vi "Autonomous Independent.vi"() -> ()   [LabVIEW 2012]
doc: "This VI is called when autonomous begins, and will automatically be terminated when autonomous ends. You can carry out timed or sensor driven robot movement independently without needing to return to the caller."
uses:
  <vilib>/Rock Robotics/WPI/DriverStation/WPI_DriverStationMatch Info.ctl
  <vilib>/Rock Robotics/WPI/Solenoid/WPI_SolenoidValue.ctl
  <vilib>/Rock Robotics/WPI/Relay/WPI_RelayValue.ctl
  Robot Global Data.vi
  <vilib>/addons/control/pid/pid.llb/PID (DBL).vi
  <vilib>/Rock Robotics/WPI/Solenoid/WPI_SolenoidSetEnum.vi
  <vilib>/Rock Robotics/WPI/Joystick/WPI_JoystickGetSetRefNum.vi
  <vilib>/addons/control/pid/NI_PID_pid.lvlib
panel:
  out "Reseting constant":bool
  in  "Threshold for shooter":dbl=0.015
  out "Ready To Fire":bool
  in  "PID gains":T1={"proportional gain (Kc)"=1.0, "integral time (Ti, min)"=0.007, "derivative time (Td, min)"=0.0} {"derivative time (Td, min)" format="%.3f"; "integral time (Ti, min)" format="%.3f"; "proportional gain (Kc)" format="%.3f"}
  in  "Maximum Encoder speed":dbl=25000.0
  out "Time Last Fired":dbl
  in  "Posistioned":string="Nothing"
  in  "S On Time":dbl=200.0
  in  "S Off Time":dbl=500.0
  in  "Shooter Speed":dbl format="%.2f"
  in  "Shooter On":bool=TRUE
  in  "Match Info":T2={"Autonomous Elapsed Seconds"=0.0, "TeleOp Elapsed Seconds"=0.0, "Disabled Elapsed Seconds"=0.0, "Visited Autonomous"=FALSE, "Visited TeleOp"=FALSE, "Visited Disabled"=FALSE, "Autonomous Settings"={"Autonomous Style"=enum."Independent", "VI Refnum"=refnum}}
  out "Angle Target":dbl
  out "Distance From Target":dbl
  in  "Current Status":string="Roaming"
  in  "Angle to Move":dbl format="%.2f"
  in  "Feet To Move at Begin":dbl format="%.2f"
  # "Be sure to right-click and choose Data Operations>>Make Current Value default if you want to save the array values with the VI"
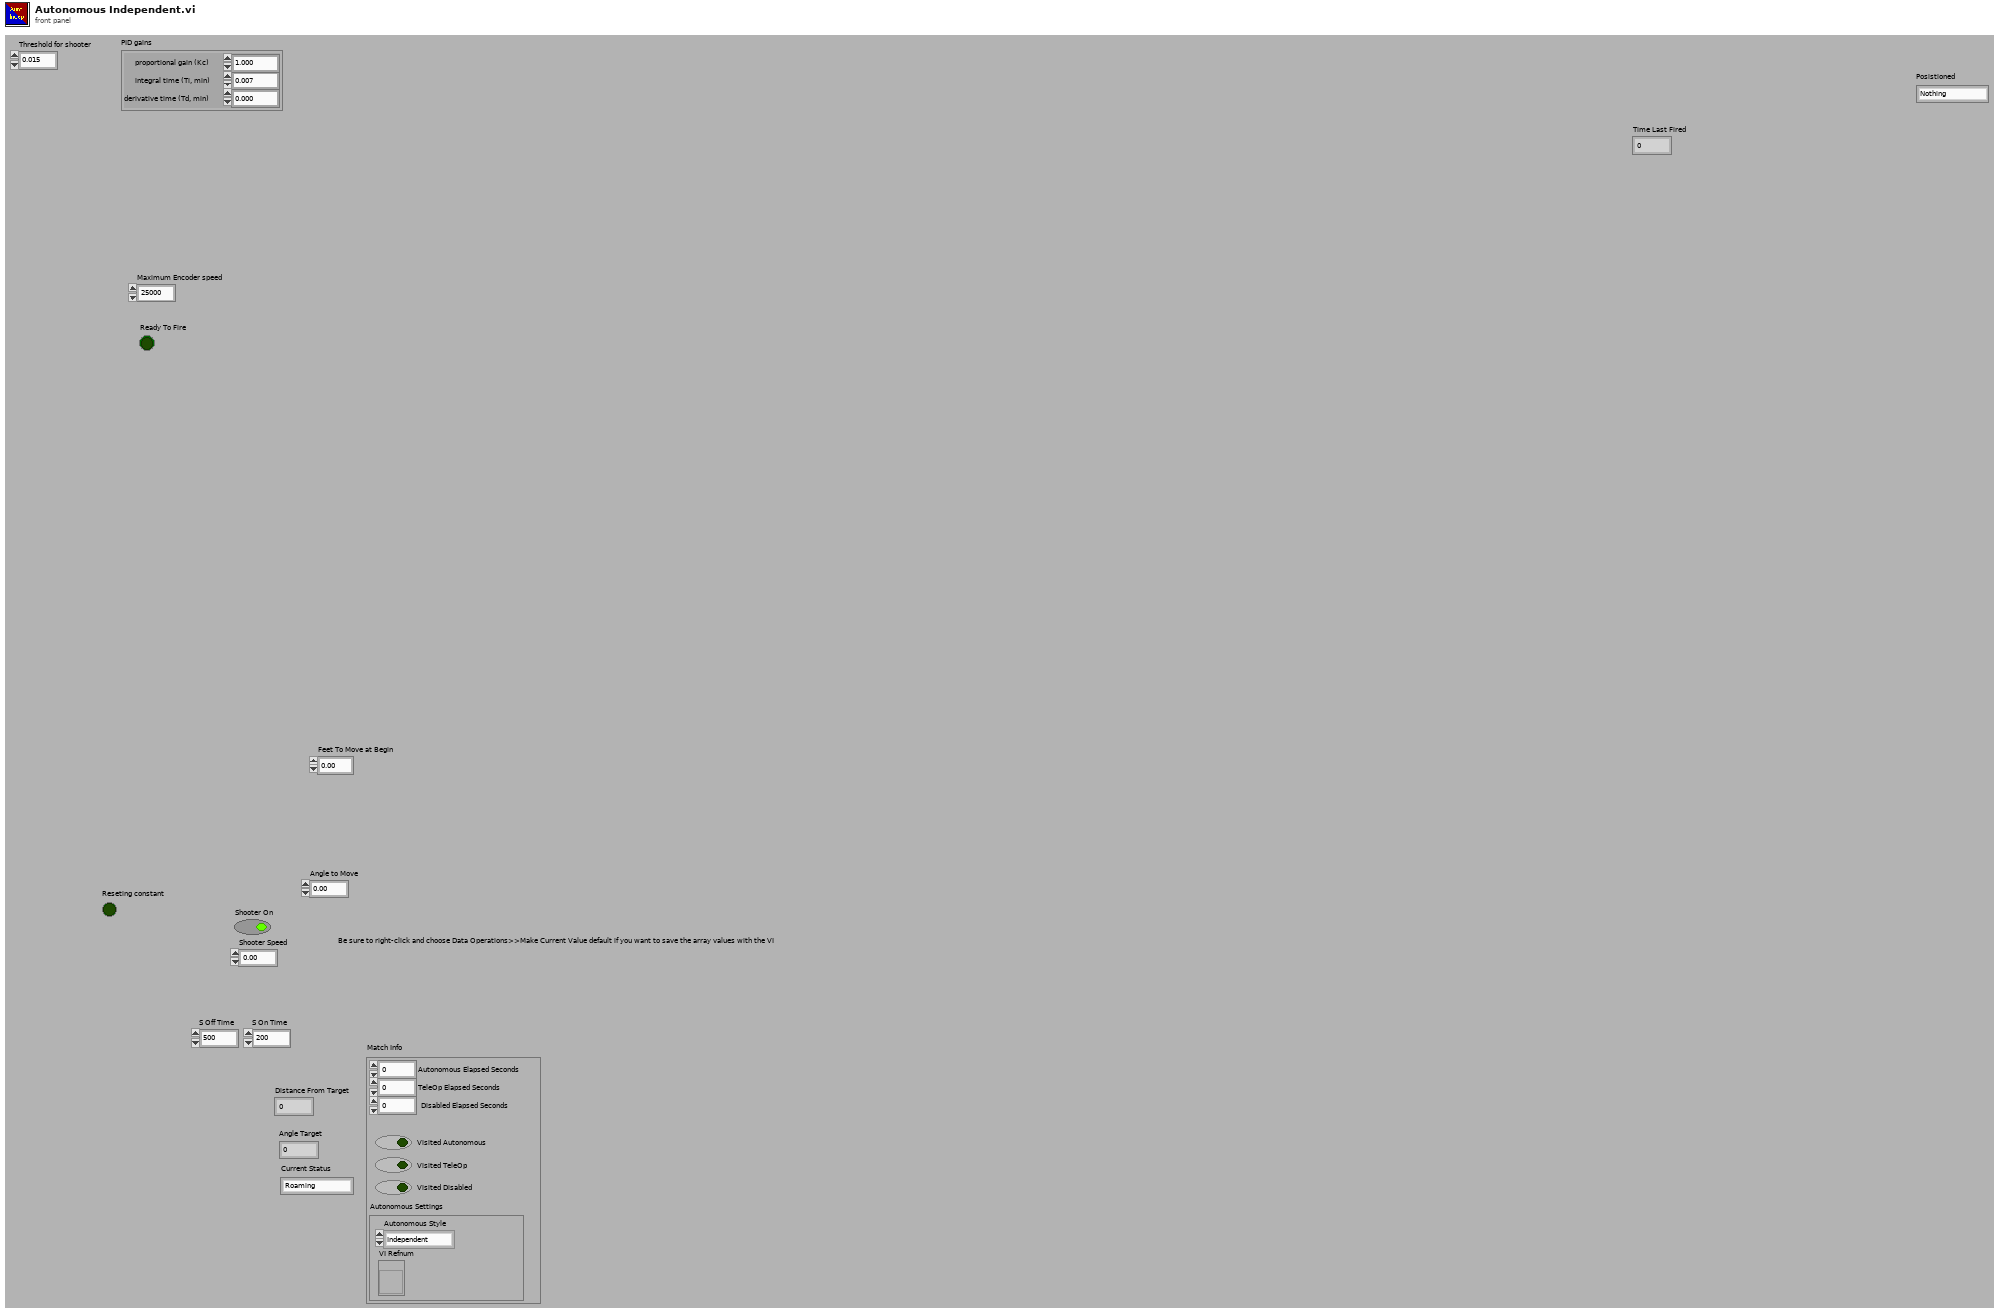
[diagram p1: front panel]
types:
  T1 = cluster{"proportional gain (Kc)":dbl, "integral time (Ti, min)":dbl, "derivative time (Td, min)":dbl}
  T2 = typedef "WPI_DriverStationMatch Info.ctl" = cluster{"Autonomous Elapsed Seconds":dbl, "TeleOp Elapsed Seconds":dbl, "Disabled Elapsed Seconds":dbl, "Visited Autonomous":bool, "Visited TeleOp":bool, "Visited Disabled":bool, "Autonomous Settings":cluster{"Autonomous Style":enum16{"Iterative", "Independent"}, "VI Refnum":refnum<vi>}}
  T3 = typedef "WPI_SolenoidValue.ctl" = enum16{"Off", "On", "Forward", "Reverse"}
  T4 = typedef "WPI_RelayValue.ctl" = enum16{"Off", "On", "Forward", "Reverse"}
  T5 = typedef "WPI_EncoderDevRef.ctl" = cluster{"DevStatus":errorcluster, "EncoderIndex":T6, "CounterIndex":T7, "DistancePerCount":dbl, "Decoding Type":T8}
  T6 = typedef "FPGA_EncoderIdx.ctl" = enum8{"Enc 0", "Enc 1", "Enc 2", "Enc 3", "Invalid"}
  T7 = typedef "FPGA_CounterCtrSystemIndex.ctl" = enum8{"Ctr 0", "Ctr 1", "Ctr 2", "Ctr 3", "Ctr 4", "Ctr 5", "Ctr 6", "Ctr 7", "Invalid"}
  T8 = typedef "WPI_EncoderType.ctl" = enum16{"1x", "2x", "4x"}
  T9 = typedef "WPI_RelayDevRef.ctl" = cluster{"DevStatus":errorcluster, "Relay Channel":T10, "Digital Module":T11, "Relay Direction":T12}
  T10 = typedef "FPGA_DIORelayChannel.ctl" = enum8{"Relay 1", "Relay 2", "Relay 3", "Relay 4", "Relay 5", "Relay 6", "Relay 7", "Relay 8", "Invalid"}
  T11 = typedef "FPGA_TypedefDigitalModule.ctl" = enum16{"Digital Module 1", "Digital Module 2"}
  T12 = typedef "WPI_RelayDirection.ctl" = enum16{"Both directions", "Forward only", "Reverse only"}
  T13 = typedef "WPI_SolenoidDevRef.ctl" = cluster{"DevStatus":errorcluster, "Solenoid Module":T14, "Forward Solenoid Channel":T15, "Reverse Solenoid Channel":T15}
  T14 = typedef "FPGA_TypedefSolenoidModule.ctl" = enum16{"Solenoid Module 1", "Solenoid Module 2"}
  T15 = typedef "WPI_SolenoidChannel.ctl" = enum8{"Solenoid 1", "Solenoid 2", "Solenoid 3", "Solenoid 4", "Solenoid 5", "Solenoid 6", "Solenoid 7", "Solenoid 8", "Invalid"}
  T16 = cluster{"Center Position":cluster{"X":dbl, "Y":dbl}, "Distance (ft)":dbl, "Center":bool}[]
  T17 = cluster{"Center Position":cluster{"X":dbl, "Y":dbl}, "Distance (ft)":dbl, "Center":bool}
  T18 = typedef "WPI_MotorControlDeviceRef.ctl" = cluster{"DeviceStatus":errorcluster, "Type":enum16{"PWM", "CAN"}, "PWM":cluster{"Digital Module":T11, "PWM Channel":T19, "DeadBand":T20}, "CAN":cluster{"Device Number":u8, "Control Mode":T21, "Semaphore":T22, "Max Vout":dbl}, "Invert":bool, "TransformRef":T23, "InvTransformRef":T23}
  T19 = typedef "FPGA_DIOPWMChannel.ctl" = enum8{"PWM 1", "PWM 2", "PWM 3", "PWM 4", "PWM 5", "PWM 6", "PWM 7", "PWM 8", "PWM 9", "PWM 10", "Invalid"}
  T20 = typedef "WPI_PWMDeadband.ctl" = cluster{"Name":string, "maxPositivePwm":i32, "minPositivePwm":i32, "centerPwm":i32, "maxNegativePwm":i32, "minNegativePwm":i32, "angularRange":u16}
  T21 = typedef "WPI_CANJaguar_ControlMode.ctl" = enum8{"Percent VBus", "Current", "Speed", "Position", "Voltage"}
  T22 = typedef "Semaphore RefNum" = refnum<k1>
  T23 = typedef "WPI_PWMTransform_ConPane.ctl" = refnum<vi>
  T24 = typedef "WPI_JoystickDevRef.ctl" = cluster{"Device":T25}
  T25 = typedef "WPI_JoystickDeviceEnum.ctl" = enum16{"USB 1", "USB 2", "USB 3", "USB 4", "Kinect 1", "Kinect 2"}
  T26 = cluster{"axis 1 (x)":dbl, "axis 2 (y)":dbl, "axis 3 (throttle)":dbl, "axis 4":dbl, "axis 5":dbl, "axis 6":dbl}
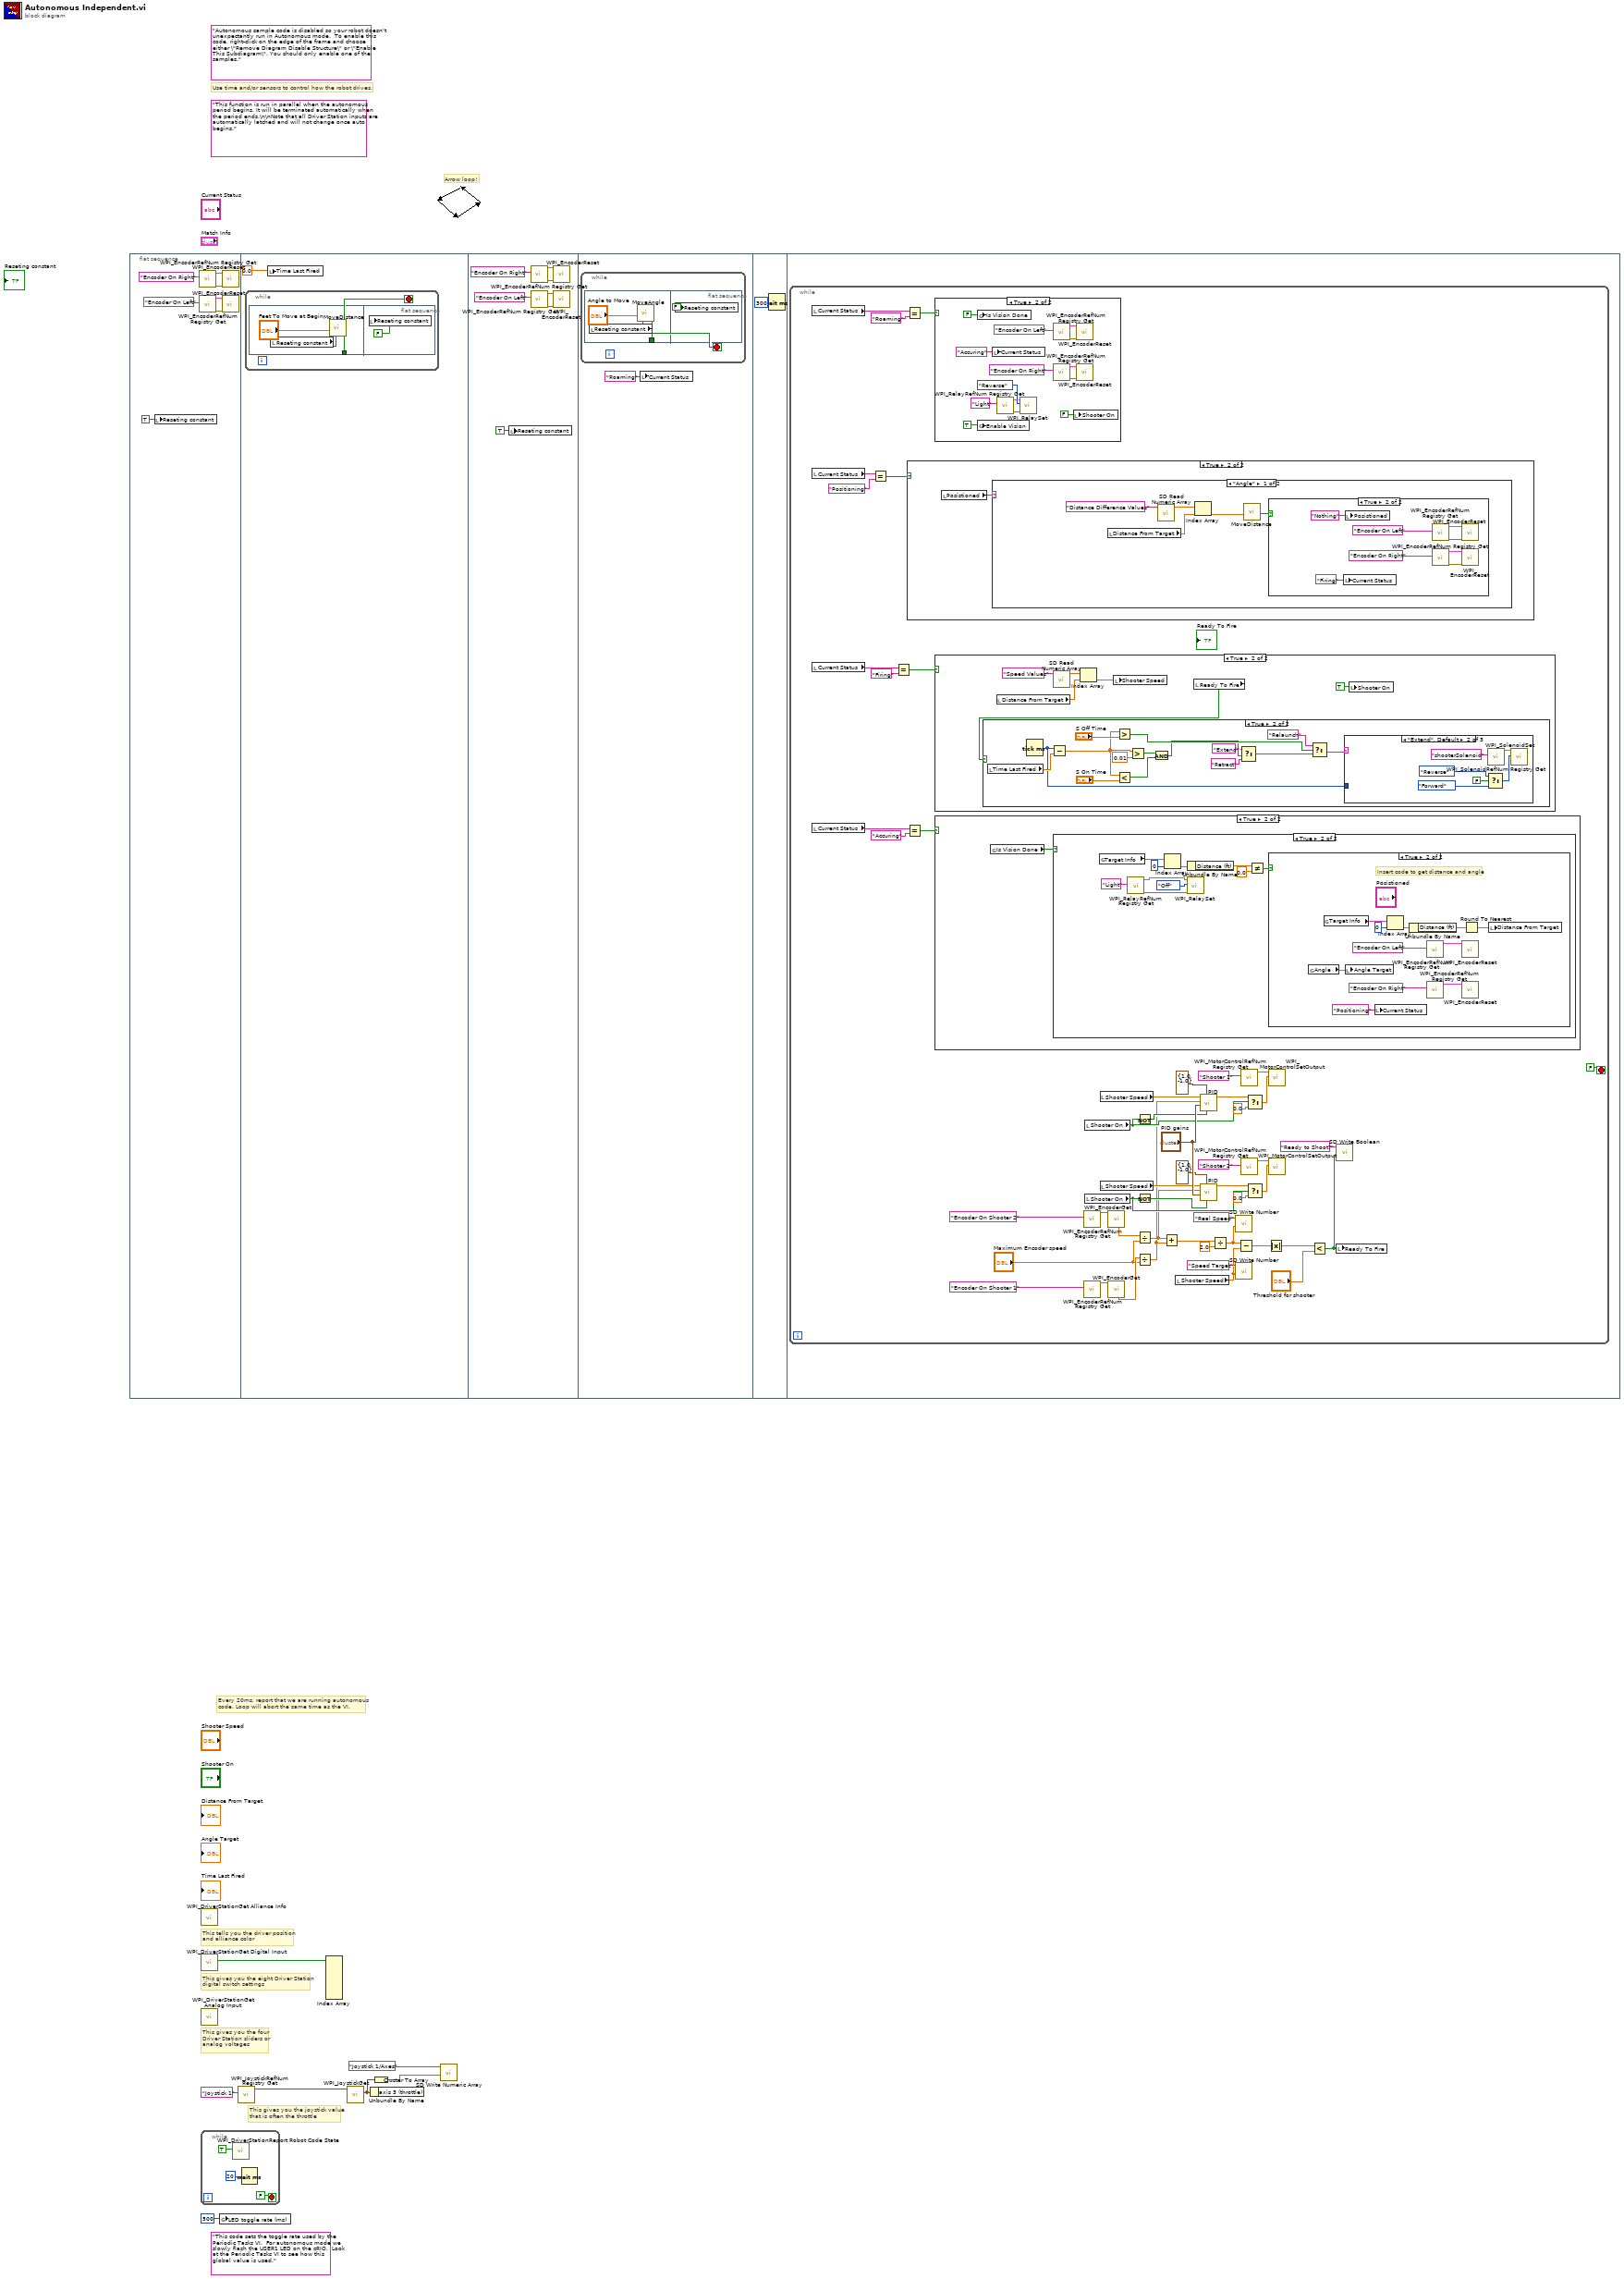
[diagram p0: block diagram]
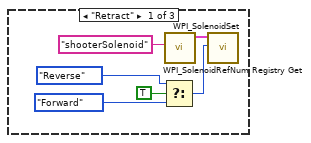
[diagram p4: hidden frame]
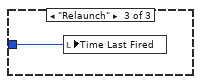
[diagram p5: hidden frame]
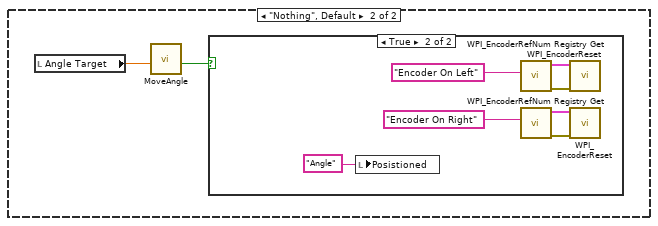
[diagram p9: hidden frame]
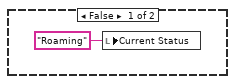
[diagram p13: hidden frame]
diagram:
  (unwired) "This code sets the toggle rate used by the Periodic Tasks VI.  For autonomous mode we slowly flash the USER1 LED on the cRIO.  Look at the Periodic Tasks VI to see how this global value is used."
  (unwired) "Autonomous sample code is disabled so your robot doesn't unexpectantly run in Autonomous mode.  To enable this code, right-click on the edge of the frame and choose either \"Remove Diagram Disable Structure\" or \"Enable This Subdiagram\". You should only enable one of the samples."
  (unwired) "This function is run in parallel when the autonomous period begins. It will be terminated automatically when the period ends.\n\nNote that all Driver Station inputs are automatically latched and will not change once auto begins."
  # "Arrow loop!"
  # "Every 20ms, report that we are running autonomous\ncode. Loop will abort the same time as the VI."
  # "This gives you the joystick value\nthat is often the throttle"
  # "Use time and/or sensors to control how the robot drives."
  # "This tells you the driver position\nand alliance color"
  # "This gives you the eight Driver Station\ndigital switch settings"
  # "This gives you the four\nDriver Station sliders or\nanalog voltages"
  n1 = flat-sequence {
    frame #0 {
      n2 = local write "Reseting constant"(TRUE ("Reseting constant")) -> ()
      n3 = call <vilib>:"WPI_EncoderRefNum Registry Get.vi"("refnum name"="Encoder On Right") -> ("error out"=w9:errorcluster, "EncoderDevRef"=w10:T5)  [unwired: 9 in]
      n4 = call <vilib>:"WPI_EncoderRefNum Registry Get.vi"("refnum name"="Encoder On Left") -> ("error out"=w11:errorcluster, "EncoderDevRef"=w12:T5)  [unwired: 9 in]
      n5 = call <vilib>:"WPI_EncoderReset.vi"("error in (no error)"=w9, "EncoderDevRef"=w10) -> ()  [unwired: 8 in, 2 out]
      n6 = call <vilib>:"WPI_EncoderReset.vi"("error in (no error)"=w11, "EncoderDevRef"=w12) -> ()  [unwired: 8 in, 2 out]
    }
    frame #1 {
      n7 = while {
        stop <- w16 stop-if-true
        n8 = flat-sequence {
          tunnel: [w19] -> w16
          frame #0 {
            n9 = local read "Reseting constant"() -> (w17:bool)
            n10 = call "MoveDistance.vi"("reinitialize? (F)"=w17, "Distance From Target"="Feet To Move at Begin") -> ("Done?"=w19:bool)  [unwired: 9 in]
          }
          frame #1 {
            n11 = local write "Reseting constant"(FALSE ("Reseting constant")) -> ()
          }
        }
      }
      n12 = local write "Time Last Fired"(0.0 ("Time Last Fired")) -> ()
    }
    frame #2 {
      n13 = local write "Reseting constant"(TRUE ("Reseting constant")) -> ()
      n14 = call <vilib>:"WPI_EncoderRefNum Registry Get.vi"("refnum name"="Encoder On Right") -> ("error out"=w27:errorcluster, "EncoderDevRef"=w26:T5)  [unwired: 9 in]
      n15 = call <vilib>:"WPI_EncoderRefNum Registry Get.vi"("refnum name"="Encoder On Left") -> ("error out"=w25:errorcluster, "EncoderDevRef"=w24:T5)  [unwired: 9 in]
      n16 = call <vilib>:"WPI_EncoderReset.vi"("error in (no error)"=w27, "EncoderDevRef"=w26) -> ()  [unwired: 8 in, 2 out]
      n17 = call <vilib>:"WPI_EncoderReset.vi"("error in (no error)"=w25, "EncoderDevRef"=w24) -> ()  [unwired: 8 in, 2 out]
    }
    frame #3 {
      n18 = while {
        stop <- w29 stop-if-true
        n19 = flat-sequence {
          tunnel: [w31] -> w29
          frame #0 {
            n20 = local read "Reseting constant"() -> (w30:bool)
            n21 = call "MoveAngle.vi"("reinitialize? (F)"=w30, "Angle Target"="Angle to Move") -> ("Done?"=w31:bool)  [unwired: 9 in]
          }
          frame #1 {
            n22 = local write "Reseting constant"(FALSE ("Reseting constant")) -> ()
          }
        }
      }
      n23 = local write "Current Status"("Roaming" ("Current Status")) -> ()
    }
    frame #4 {
      n24 = Wait (ms)(milliseconds to wait=u32 300) -> ()  [unwired: 1 out]
    }
    frame #5 {
      n25 = while {
        stop <- FALSE stop-if-true
        n26 = local read "Current Status"() -> (w78:string)
        n27 = local read "Current Status"() -> (w82:string)
        n28 = local read "Current Status"() -> (w75:string)
        n29 = local read "Current Status"() -> (w86:string)
        n30 = Equal?(x=w82, y="Positioning") -> (x = y?=w80:bool)
        n31 = Equal?(x=w75, y="Firing") -> (x = y?=w76:bool)
        n32 = Equal?(x=w78, y="Roaming") -> (x = y?=w77:bool)
        n33 = Equal?(x=w86, y="Accuring") -> (x = y?=w84:bool)
        n34 = case shown="True" w80 {
          frame False {
          }
          frame True {
            n35 = local read "Posistioned"() -> (w135:string)
            n36 = case shown="\"Angle\"" w135 {
              frame "Angle" {
                n37 = local read "Distance From Target"() -> (w138:dbl)
                n38 = call <vilib>:"SD Read Numeric Array.vi"("Name"="Distance Difference Values") -> ("Numeric Array"=w140:dbl[])  [unwired: 8 in, 2 out]
                n39 = Index Array(array=w140, index=w138) -> (element=w137:dbl)
                n40 = call "MoveDistance.vi"("Distance From Target"=w137) -> ("Done?"=w136:bool)  [unwired: 10 in]
                n41 = case shown="True" w136 {
                  frame False {
                  }
                  frame True {
                    n42 = local write "Current Status"("Firing" ("Current Status")) -> ()
                    n43 = local write "Posistioned"("Nothing" ("Posistioned")) -> ()
                    n44 = call <vilib>:"WPI_EncoderRefNum Registry Get.vi"("refnum name"="Encoder On Left") -> ("error out"=w144:errorcluster, "EncoderDevRef"=w145:T5)  [unwired: 9 in]
                    n45 = call <vilib>:"WPI_EncoderRefNum Registry Get.vi"("refnum name"="Encoder On Right") -> ("error out"=w146:errorcluster, "EncoderDevRef"=w147:T5)  [unwired: 9 in]
                    n46 = call <vilib>:"WPI_EncoderReset.vi"("error in (no error)"=w144, "EncoderDevRef"=w145) -> ()  [unwired: 8 in, 2 out]
                    n47 = call <vilib>:"WPI_EncoderReset.vi"("error in (no error)"=w146, "EncoderDevRef"=w147) -> ()  [unwired: 8 in, 2 out]
                  }
                }
              }
              frame "Nothing", Default {
                n48 = local read "Angle Target"() -> (w150:dbl)
                n49 = call "MoveAngle.vi"("Angle Target"=w150) -> ("Done?"=w149:bool)  [unwired: 10 in]
                n50 = case shown="True" w149 {
                  frame False {
                  }
                  frame True {
                    n51 = local write "Posistioned"("Angle" ("Posistioned")) -> ()
                    n52 = call <vilib>:"WPI_EncoderRefNum Registry Get.vi"("refnum name"="Encoder On Left") -> ("error out"=w155:errorcluster, "EncoderDevRef"=w154:T5)  [unwired: 9 in]
                    n53 = call <vilib>:"WPI_EncoderRefNum Registry Get.vi"("refnum name"="Encoder On Right") -> ("error out"=w153:errorcluster, "EncoderDevRef"=w152:T5)  [unwired: 9 in]
                    n54 = call <vilib>:"WPI_EncoderReset.vi"("error in (no error)"=w155, "EncoderDevRef"=w154) -> ()  [unwired: 8 in, 2 out]
                    n55 = call <vilib>:"WPI_EncoderReset.vi"("error in (no error)"=w153, "EncoderDevRef"=w152) -> ()  [unwired: 8 in, 2 out]
                  }
                }
              }
            }
          }
        }
        n56 = case shown="True" w77 {
          frame False {
          }
          frame True {
            n57 = global write "Robot Global Data.vi" "Is Vision Done"(FALSE ("Is Vision Done")) -> ()
            n58 = global write "Robot Global Data.vi" "Enable Vision"(TRUE ("Enable Vision")) -> ()
            n59 = local write "Current Status"("Accuring" ("Current Status")) -> ()
            n60 = call <vilib>:"WPI_RelayRefNum Registry Get.vi"("refnum name"="Light") -> ("error out"=w132:errorcluster, "RelayDevRef"=w131:T9)  [unwired: 9 in]
            n61 = call <vilib>:"WPI_RelaySet.vi"("error in (no error)"=w132, "RelayValue"=WPI_RelayValue."Reverse", "RelayDevRef"=w131) -> ()  [unwired: 7 in, 2 out]
            n62 = call <vilib>:"WPI_EncoderRefNum Registry Get.vi"("refnum name"="Encoder On Left") -> ("error out"=w126:errorcluster, "EncoderDevRef"=w125:T5)  [unwired: 9 in]
            n63 = call <vilib>:"WPI_EncoderRefNum Registry Get.vi"("refnum name"="Encoder On Right") -> ("error out"=w128:errorcluster, "EncoderDevRef"=w127:T5)  [unwired: 9 in]
            n64 = local write "Shooter On"(FALSE ("Shooter On")) -> ()
            n65 = call <vilib>:"WPI_EncoderReset.vi"("error in (no error)"=w126, "EncoderDevRef"=w125) -> ()  [unwired: 8 in, 2 out]
            n66 = call <vilib>:"WPI_EncoderReset.vi"("error in (no error)"=w128, "EncoderDevRef"=w127) -> ()  [unwired: 8 in, 2 out]
          }
        }
        n67 = case shown="True" w76 {
          frame False {
          }
          frame True {
            n68 = local read "Distance From Target"() -> (w89:dbl)
            n69 = call <vilib>:"SD Read Numeric Array.vi"("Name"="Speed Values") -> ("Numeric Array"=w91:dbl[])  [unwired: 8 in, 2 out]
            n70 = Index Array(array=w91, index=w89) -> (element=w90:dbl)
            n71 = local write "Shooter Speed"(w90) -> ()
            n72 = local read "Ready To Fire"() -> (w88:bool)
            n73 = case shown="True" w88 {
              frame False {
              }
              frame True {
                n74 = local read "Time Last Fired"() -> (w107:dbl)
                n75 = Tick Count (ms)() -> (millisecond timer value=w95:u32)
                n76 = Subtract(x=w95, y=w107) -> (x-y=w100:dbl)
                n77 = Greater?(x=w100, y="S Off Time") -> (0:w103:bool)
                n78 = Less?(x=w100, y="S On Time") -> (x < y?=w97:bool)
                n79 = Greater?(x=w100, y=0.01) -> (0:w98:bool)
                n80 = And(x=w98, y=w97) -> (x .and. y?=w96:bool)
                n81 = Select(t="Extend" ("f"), s=w96, f="Retract") -> (s? t:f=w101:string)
                n82 = Select(t="Relaunch" ("f"), s=w103, f=w101) -> (s? t:f=w105:string)
                n83 = case shown="\"Extend\", Default" w105 {
                  tunnel: w95 -> [_ _ w120]
                  frame "Retract" {
                    n84 = Select(t=WPI_SolenoidValue."Reverse" ("Value"), s=TRUE, f=WPI_SolenoidValue."Forward" ("Value")) -> (s? t:f=w112:T3)
                    n85 = call <vilib>:"WPI_SolenoidRefNum Registry Get.vi"("refnum name"="shooterSolenoid") -> ("SolenoidDevRef"=w108:T13)  [unwired: 9 in, 1 out]
                    n86 = call-poly <vilib>:"WPI_SolenoidSet.vi"("Value"=w112, "SolenoidDevRef"=w108) -> ()  [unwired: 8 in, 2 out]
                  }
                  frame "Extend", Default {
                    n87 = Select(t=WPI_SolenoidValue."Reverse" ("Value"), s=FALSE, f=WPI_SolenoidValue."Forward" ("Value")) -> (s? t:f=w118:T3)
                    n88 = call <vilib>:"WPI_SolenoidRefNum Registry Get.vi"("refnum name"="shooterSolenoid") -> ("SolenoidDevRef"=w114:T13)  [unwired: 9 in, 1 out]
                    n89 = call-poly <vilib>:"WPI_SolenoidSet.vi"("Value"=w118, "SolenoidDevRef"=w114) -> ()  [unwired: 8 in, 2 out]
                  }
                  frame "Relaunch" {
                    n90 = local write "Time Last Fired"(w120) -> ()
                  }
                }
              }
            }
            n91 = local write "Shooter On"(TRUE ("Shooter On")) -> ()
          }
        }
        n92 = case shown="True" w84 {
          frame False {
          }
          frame True {
            n93 = global read "Robot Global Data.vi" "Is Vision Done"() -> (w158:bool)
            n94 = case shown="True" w158 {
              frame False {
              }
              frame True {
                n95 = global read "Robot Global Data.vi" "Target Info"() -> (w168:T16)
                n96 = call <vilib>:"WPI_RelayRefNum Registry Get.vi"("refnum name"="Light") -> ("error out"=w161:errorcluster, "RelayDevRef"=w162:T9)  [unwired: 9 in]
                n97 = Index Array(array=w168, index=0) -> (element=w166:T17)
                n98 = Unbundle By Name(w166) -> ("Distance (ft)"=w164:dbl)
                n99 = call <vilib>:"WPI_RelaySet.vi"("error in (no error)"=w161, "RelayValue"=WPI_RelayValue."Off", "RelayDevRef"=w162) -> ()  [unwired: 7 in, 2 out]
                n100 = Not Equal?(x=w164, y=0.0) -> (x != y?=w165:bool)
                n101 = case shown="True" w165 {
                  frame False {
                    n102 = local write "Current Status"("Roaming" ("Current Status")) -> ()
                  }
                  frame True {
                    # "Insert code to get distance and angle"
                    n103 = global read "Robot Global Data.vi" "Angle"() -> (w175:dbl)
                    n104 = global read "Robot Global Data.vi" "Target Info"() -> (w174:T16)
                    n105 = local write "Angle Target"(w175) -> ()
                    n106 = local write "Current Status"("Positioning" ("Current Status")) -> ()
                    n107 = Index Array(array=w174, index=0) -> (element=w172:T17)
                    n108 = Unbundle By Name(w172) -> ("Distance (ft)"=w171:dbl)
                    n109 = call <vilib>:"WPI_EncoderRefNum Registry Get.vi"("refnum name"="Encoder On Left") -> ("EncoderDevRef"=w178:T5)  [unwired: 9 in, 1 out]
                    n110 = call <vilib>:"WPI_EncoderRefNum Registry Get.vi"("refnum name"="Encoder On Right") -> ("EncoderDevRef"=w177:T5)  [unwired: 9 in, 1 out]
                    n111 = call <vilib>:"WPI_EncoderReset.vi"("EncoderDevRef"=w178) -> ()  [unwired: 9 in, 2 out]
                    n112 = call <vilib>:"WPI_EncoderReset.vi"("EncoderDevRef"=w177) -> ()  [unwired: 9 in, 2 out]
                    n113 = Round To Nearest(number=w171) -> (nearest integer value=w170:dbl)
                    n114 = local write "Distance From Target"(w170) -> ()
                  }
                }
              }
            }
          }
        }
        n115 = call <vilib>:"WPI_EncoderRefNum Registry Get.vi"("refnum name"="Encoder On Shooter 2") -> ("EncoderDevRef"=w61:T5)  [unwired: 9 in, 1 out]
        n116 = call <vilib>:"WPI_EncoderRefNum Registry Get.vi"("refnum name"="Encoder On Shooter 1") -> ("EncoderDevRef"=w70:T5)  [unwired: 9 in, 1 out]
        n117 = local read "Shooter On"() -> (w50:bool)
        n118 = local read "Shooter On"() -> (w51:bool)
        n119 = local read "Shooter Speed"() -> (w49:dbl)
        n120 = local read "Shooter Speed"() -> (w48:dbl)
        n121 = call <vilib>:"WPI_EncoderGet.vi"("EncoderDevRef"=w61) -> ("Rate"=w53:dbl)  [unwired: 5 in, 5 out]
        n122 = call <vilib>:"WPI_EncoderGet.vi"("EncoderDevRef"=w70) -> ("Rate"=w54:dbl)  [unwired: 5 in, 5 out]
        n123 = Not(x=w50) -> (.not. x?=w72:bool)
        n124 = Not(x=w51) -> (.not. x?=w63:bool)
        n125 = Divide(x=w53, y="Maximum Encoder speed") -> (x/y=w46:dbl)
        n126 = Divide(x=w54, y="Maximum Encoder speed") -> (x/y=w45:dbl)
        n127 = Add(x=w46, y=w45) -> (x+y=w44:dbl)
        n128 = local read "Shooter Speed"() -> (w41:dbl)
        n129 = call-poly <vilib>:"PID.vi"("reinitialize? (F)"=w72, "output range"=cluster{"output high":dbl, "output low":dbl} {"output high"=1.0, "output low"=-1.0}, "PID gains"="PID gains", "process variable"=w45, "setpoint"=w49) -> ("output"=w71:dbl)  [unwired: 5 in, 1 out]
        n130 = call-poly <vilib>:"PID.vi"("reinitialize? (F)"=w63, "output range"=cluster{"output high":dbl, "output low":dbl} {"output high"=1.0, "output low"=-1.0}, "PID gains"="PID gains", "process variable"=w46, "setpoint"=w48) -> ("output"=w62:dbl)  [unwired: 5 in, 1 out]
        n131 = Divide(x=w44, y=2.0) -> (x/y=w40:dbl)
        n132 = call <vilib>:"SD Write Number.vi"("Numeric"=w40, "Name"="Real Speed") -> ()  [unwired: 8 in, 2 out]
        n133 = call <vilib>:"SD Write Number.vi"("Numeric"=w41, "Name"="Speed Target") -> ()  [unwired: 8 in, 2 out]
        n134 = Subtract(x=w40, y=w41) -> (x-y=w39:dbl)
        n135 = call <vilib>:"WPI_MotorControlRefNum Registry Get.vi"("refnum name"="Shooter 1") -> ("MotorControlDevRef"=w65:T18)  [unwired: 9 in, 1 out]
        n136 = call <vilib>:"WPI_MotorControlRefNum Registry Get.vi"("refnum name"="Shooter 2") -> ("MotorControlDevRef"=w56:T18)  [unwired: 9 in, 1 out]
        n137 = Select(t=w71, s=w50, f=0.0) -> (s? t:f=w67:dbl)
        n138 = Select(t=w62, s=w51, f=0.0) -> (s? t:f=w58:dbl)
        n139 = Absolute Value(x=w39) -> (abs(x)=w38:dbl)
        n140 = call <vilib>:"WPI_MotorControlSetOutput.vi"("Output"=w67, "MotorControlDevRef"=w65) -> ()  [unwired: 7 in, 3 out]
        n141 = call <vilib>:"WPI_MotorControlSetOutput.vi"("Output"=w58, "MotorControlDevRef"=w56) -> ()  [unwired: 7 in, 3 out]
        n142 = Less?(x=w38, y="Threshold for shooter") -> (x < y?=w36:bool)
        n143 = call <vilib>:"SD Write Boolean.vi"("Boolean"=w36, "Name"="Ready to Shoot?") -> ()  [unwired: 8 in, 2 out]
        n144 = local write "Ready To Fire"(w36) -> ()
      }
    }
  }
  n145 = call <vilib>:"WPI_DriverStationGet Alliance Info.vi"() -> ()  [unwired: 12 out]
  n146 = call <vilib>:"WPI_DriverStationGet Digital Input.vi"() -> ("Driver Station Digital Input (1-8)"=w7:bool[])  [unwired: 11 out]
  n147 = call <vilib>:"WPI_DriverStationGet Analog Input.vi"() -> ()  [unwired: 12 out]
  n148 = while {
    stop <- FALSE stop-if-true
    n149 = call <vilib>:"WPI_DriverStationReport Robot Code State.vi"("Autonomous"=TRUE) -> ()  [unwired: 10 in, 1 out]
    n150 = Wait (ms)(milliseconds to wait=u32 20) -> ()  [unwired: 1 out]
  }
  n151 = global write "Robot Global Data.vi" "LED toggle rate (ms)"(u32 500 ("LED ms toggle rate")) -> ()
  n152 = call <vilib>:"WPI_JoystickRefNum Registry Get.vi"("refnum name"="Joystick 1") -> ("JoystickDevRef"=w5:T24)  [unwired: 1 in, 9 out]
  n153 = Index Array(array=w7) -> ()  [unwired: 8 in, 8 out]
  n154 = call <vilib>:"WPI_JoystickGet.vi"("JoystickDevRef"=w5) -> ("Axes"=w2:T26)  [unwired: 1 in, 5 out]
  n155 = Unbundle By Name(w2) -> ()  [unwired: 1 out]
  n156 = Cluster To Array(cluster=w2) -> (array=w3:dbl[])
  n157 = call <vilib>:"SD Write Numeric Array.vi"("Numeric Array"=w3, "Name"="Joystick 1/Axes") -> ()  [unwired: 8 in, 2 out]
